vi "Main FK.vi"() -> ()   [LabVIEW 2017]
uses:
  <vilib>/Native 3D Graph/xcontrol/3DPC_SurfacePlot.xctl
  <vilib>/Native 3D Graph/classes/Line/Line.lvclass
  <vilib>/Platform/TimedLoop/XDataNode/timing_clust.ctl
  <vilib>/Platform/TimedLoop/XDataNode/nitl_modes.ctl
  <vilib>/Platform/TimedLoop/XDataNode/wakeup.ctl
  <vilib>/Analysis/Matrix/Datatypes/RealMatrix.ctl
  <vilib>/Utility/error.llb/DialogType.ctl
  <vilib>/Analysis/baseanly.llb/A x Vector.vi
  <vilib>/Analysis/baseanly.llb/Real A x B.vi
  <vilib>/Analysis/_algsub.llb/Vector Norm.vi
  <vilib>/Analysis/_algsub.llb/Real Vector Norm.vi
  <vilib>/Analysis/baseanly.llb/Outer Product.vi
  <vilib>/Analysis/baseanly.llb/Real Outer Product.vi
  <vilib>/robotics/Kinematics/Create Lie Group Matrix.vi
  <vilib>/Analysis/coordinate.llb/Direction Cosines To Euler Angles.vi
  <vilib>/Analysis/7linalg.llb/Create Special Matrix.vi
  <vilib>/Analysis/7linalg.llb/Create Special Real Matrix.vi
  <vilib>/Analysis/Matrix/Numeric/Multiply/Multiply.vi
  <vilib>/Analysis/Matrix/Numeric/Multiply/Multiply - RM,R.vi
  <vilib>/Analysis/Matrix/Numeric/Multiply/Multiply - R,RM.vi
  <vilib>/Analysis/Matrix/Numeric/Add/Add.vi
  <vilib>/Analysis/Matrix/Numeric/Add/Add - RM,RM.vi
  <vilib>/platform/TimedLoop/XDataNode/XDataNode.xnode
  <vilib>/robotics/Kinematics/NI_Kinematics.lvlib
  <vilib>/Analysis/NI_AALBase.lvlib
  <vilib>/Platform/TimedLoop/XDataNode/XDNodeRunTimeDep.lvlib
  <vilib>/Analysis/Matrix/NI_Matrix.lvlib
panel:
  out "FT":dbl[](array[numeric])
  out "w3c":dbl[](array[numeric])=[-0.5089191509681598, -0.8606888462607745, 0.014697200418595196]
  out "w1c":dbl[](array[numeric])=[0.9992375220058815, 0.022541625315148195, -0.031878672238615374]
  out "w2c":dbl[](array[numeric])=[-0.4945004015747698, 0.8691315050710928, 0.008931950248859025]
  out "u3":dbl[](array[numeric])=[-0.7071067811865474, 0.4082482904638634, -0.5773502691896257]
  out "u1":dbl[](array[numeric])=[0.0, -0.816496580927726, -0.5773502691896257]
  out "u2":dbl[](array[numeric])=[0.7071067811865476, 0.40824829046386285, -0.5773502691896257]
  in  "radius":dbl=1.0
  in  "damping":dbl[](array[numeric])=[0.5, 0.5, 0.5]
  out "3D Graph":refnum<class "Base Datatype.lvclass">[](xcontrol)
  in  "theta0":dbl[](array[numeric])=[0.0, 0.0, 0.0] format="%#_15g"
  in  "Kd":dbl=0.01 format="%#_13g"
  in  "Kp":dbl=10.0 format="%#_13g"
  out "thetac":dbl[](array[numeric])=[-0.03905316656235388, 0.010939578455381647, 0.018001293030222833] format="%#_15g"
  out "v3c":dbl[](array[numeric])=[0.5535037631925916, -0.3402635412966427, -0.7601672885595036]
  out "v1c":dbl[](array[numeric])=[-0.03873377001737612, 0.6749587725327184, -0.7368380761343479]
  out "v2c":dbl[](array[numeric])=[-0.6206923298860185, -0.34591671533767604, -0.7036211037701037]
  out "beta2":dbl=0.7460127831658564
  out "v30":dbl[](array[numeric])=[0.5877852522924729, -0.33935797363675174, -0.7344008870614411]
  out "v10":dbl[](array[numeric])=[0.0, 0.6787159472735029, -0.7344008870614411]
  out "v20":dbl[](array[numeric])=[-0.5877852522924731, -0.3393579736367513, -0.7344008870614411]
  out "dt":dbl=0.001
  in  "Period":i64=1
  out "v2d":dbl[](array[numeric])=[-0.6305174466734633, -0.34790000489268624, -0.6938395607314696]
  out "v1d":dbl[](array[numeric])=[-0.050680478981355706, 0.673803235637673, -0.7371707323913453]
  out "v3d":dbl[](array[numeric])=[0.5427020452710659, -0.34055660320835135, -0.7677862268039098]
  out "thetad":dbl[](array[numeric])=[-0.0511004594719751, 0.014220574258536452, 0.023656720268484584] format="%#_15g"
  out "message":string="No Error"
  out "error?":bool
  in  "stop":bool
  out "beta1":dbl=0.9553166181245093
  out "gamma2":dbl=1.2566370614359172
  out "gamma1":dbl=1.5707963267948966
  out "alpha2":dbl=1.5707963267948966
  out "alpha1":dbl=1.5707963267948966
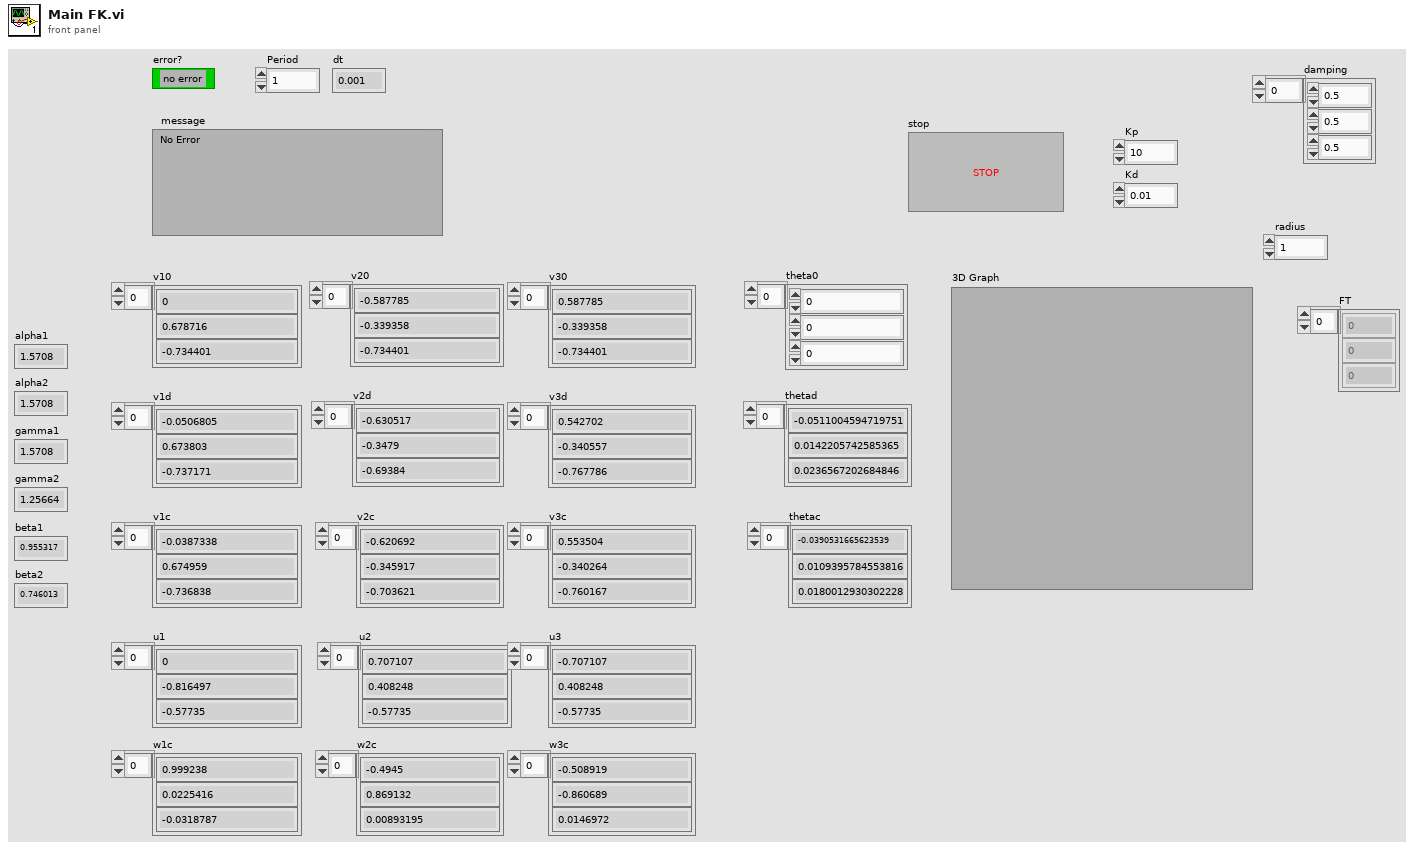
[diagram p1: front panel]
types:
  T1 = typedef "XDNodeRunTimeDep.lvlib/timing_clust.ctl" = cluster{"Expected End [f-1]":u64, "Actual End [f-1]":u64, "Finished Late? [f-1]":bool, "Expected End [i-1]":u64, "Actual End [i-1]":u64, "Finished Late? [i-1]":bool, "Expected Start [i]":u64, "Actual Start [i]":u64, "Expected Start [f]":u64, "Actual Start [f]":u64, "Source Name":string, "Structure Name":string, "Period":i64, "Deadline":i64, "Offset":i64, "Start":i64, "Priority":i32, "Timeout":i32, "Mode":T2, "Wakeup Reason":T3, "Error":errorcluster, "Source Type":string, "Secondary Source Type":string, "Global End Time":u64, "Global Start Time":u64, "Frame Duration":u64, "Iteration Duration":u64, "Assigned CPU":i32, "I/O Scan Engine Mode":u32}
  T2 = typedef "XDNodeRunTimeDep.lvlib/nitl_modes.ctl" = enum32{"No Change", "Process missed periods, maintain original phase", "Discard missed periods, maintain original phase", "Process missed periods, ignore original phase", "Discard missed periods, ignore original phase"}
  T3 = typedef "XDNodeRunTimeDep.lvlib/wakeup.ctl" = enum32{"Normal", "Aborted", "Asynchronous wakeup", "Timing source error", "Timed loop error", "Timeout"}
  T4 = typedef "NI_Matrix.lvlib/RealMatrix.ctl" = dbl[][]
  T5 = typedef "DialogType.ctl" = u16
  T6 = cluster{"phi (Z)":dbl, "theta (X)":dbl, "psi (Z)":dbl}
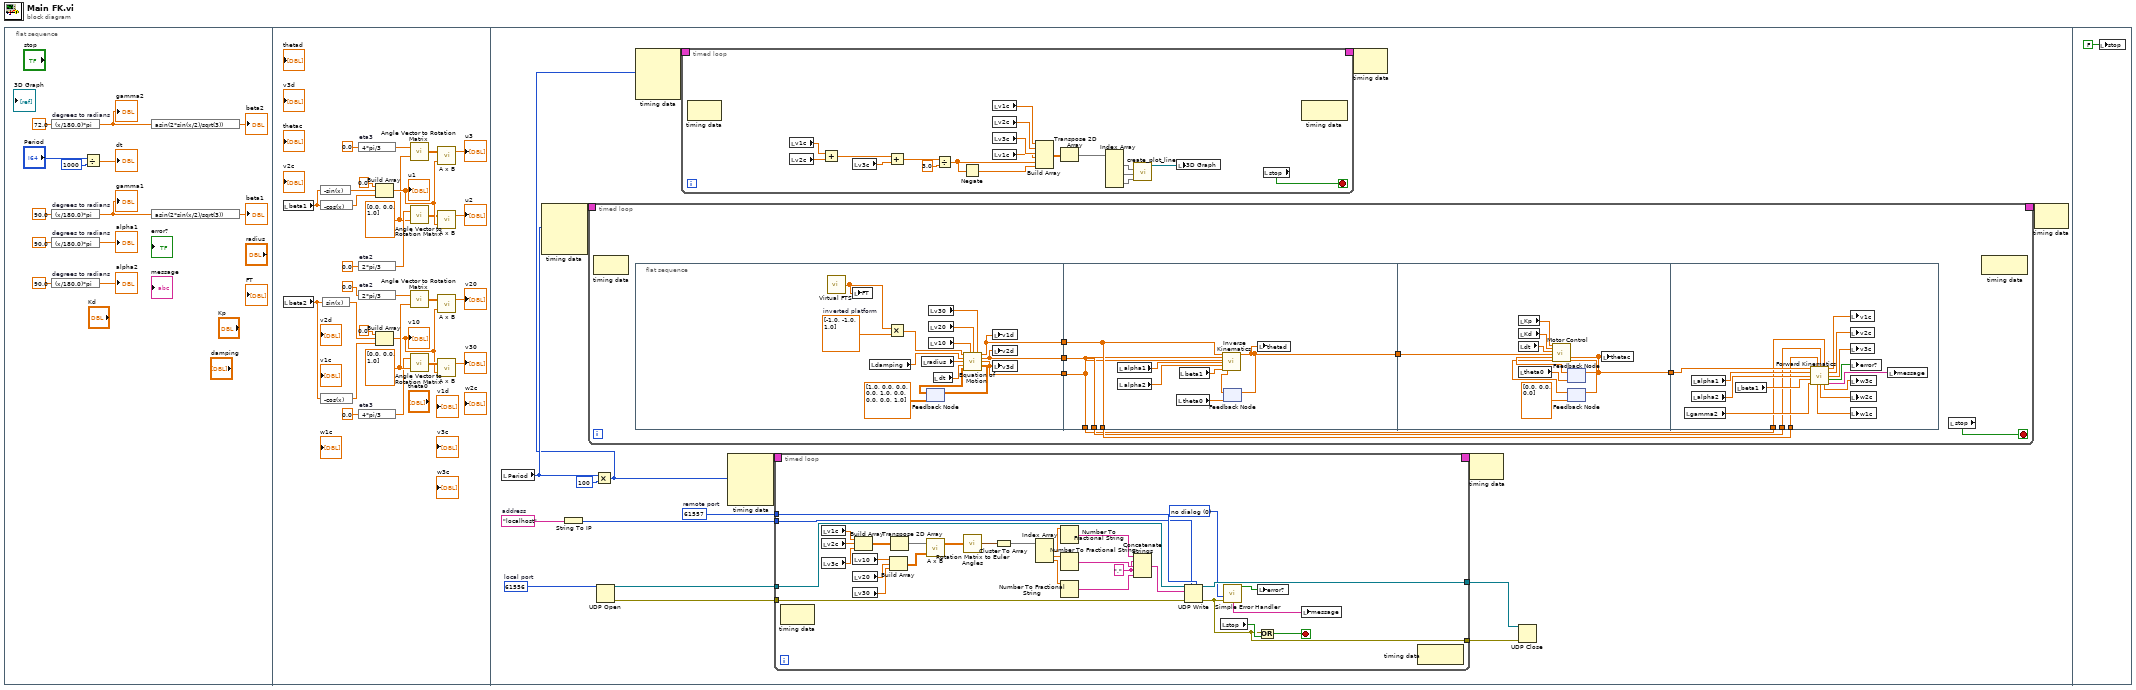
[diagram p0: block diagram]
diagram:
  n1 = flat-sequence {
    frame #0 {
      # "Design Parameters"
      n2 = expression code="(x/180.0)*pi" "degrees to radians"(72.0 ("gamma2")) -> (w5:dbl)
      "gamma2" <- w5
      n3 = expression code="(x/180.0)*pi" "degrees to radians"(90.0 ("gamma1")) -> (w7:dbl)
      "gamma1" <- w7
      n4 = expression code="(x/180.0)*pi" "degrees to radians"(90.0 ("alpha1")) -> (→"alpha1":dbl)
      n5 = expression code="(x/180.0)*pi" "degrees to radians"(90.0 ("alpha2")) -> (→"alpha2":dbl)
      n6 = Divide(x="Period", y=i64 1000) -> (x/y=→"dt":dbl)
      n7 = expression code="asin(2*sin(x/2)/sqrt(3))"(w5) -> (→"beta2":dbl)
      n8 = expression code="asin(2*sin(x/2)/sqrt(3))"(w7) -> (→"beta1":dbl)
    }
    frame #1 {
      w17 = dbl[] [0.0, 0.0, 1.0] ("vector")
      w38 = dbl[] [0.0, 0.0, 1.0] ("vector")
      # "Kinematics Variables"
      n9 = local read "beta1"() -> (w27:dbl)
      n10 = local read "beta2"() -> (w28:dbl)
      n11 = expression code="-cos(x)"(w27) -> (w16:dbl)
      n12 = expression code="-cos(x)"(w28) -> (w39:dbl)
      n13 = expression code="-sin(x)"(w27) -> (w15:dbl)
      n14 = expression code="sin(x)"(w28) -> (w40:dbl)
      n15 = expression code="4*pi/3" "eta3"(0.0) -> (w19:dbl)
      n16 = expression code="2*pi/3" "eta2"(0.0) -> (w18:dbl)
      n17 = expression code="2*pi/3" "eta2"(0.0) -> (w37:dbl)
      n18 = expression code="4*pi/3" "eta3"(0.0) -> (w36:dbl)
      n19 = Build Array(0.0 ("element"), w15, w16) -> (w24:dbl[])
      "u1" <- w24
      n20 = Build Array(0.0 ("element"), w40, w39) -> (w31:dbl[])
      "v10" <- w31
      n21 = call <vilib>:"Angle Vector to Rotation Matrix.vi"("vector"=w17, "angle"=w19) -> ("rotation matrix"=w21:T4)
      n22 = call <vilib>:"Angle Vector to Rotation Matrix.vi"("vector"=w17, "angle"=w18) -> ("rotation matrix"=w20:T4)
      n23 = call <vilib>:"Angle Vector to Rotation Matrix.vi"("vector"=w38, "angle"=w37) -> ("rotation matrix"=w35:T4)
      n24 = call <vilib>:"Angle Vector to Rotation Matrix.vi"("vector"=w38, "angle"=w36) -> ("rotation matrix"=w34:T4)
      n25 = call-poly <vilib>:"A x B.vi"("Vector"=w24, "A"=w21) -> ("A x Vector"=→"u3":dbl[])  [unwired: 1 out]
      n26 = call-poly <vilib>:"A x B.vi"("Vector"=w24, "A"=w20) -> ("A x Vector"=→"u2":dbl[])  [unwired: 1 out]
      n27 = call-poly <vilib>:"A x B.vi"("Vector"=w31, "A"=w35) -> ("A x Vector"=→"v20":dbl[])  [unwired: 1 out]
      n28 = call-poly <vilib>:"A x B.vi"("Vector"=w31, "A"=w34) -> ("A x Vector"=→"v30":dbl[])  [unwired: 1 out]
    }
    frame #2 {
      w51 = "localhost"  # address
      w52 = u16 61557  # remote port
      w49 = u16 61556  # local port
      # "FK/IK"
      n29 = local read "Period"() -> (w56:i64)
      n30 = node-c288(w56) -> (w58:T1)  [unwired: 3 in]
      n31 = String To IP(1:w51) -> (0:w50:u32)
      n32 = timed-loop {
        timing: w58 -> [_]
        timing-out: [_] -> w57
        stop <- w129 stop-if-true
        n33 = node-c288() -> ()  [unwired: 1 in, 1 out]
        n34 = flat-sequence {
          tunnel: [w135] -> w123
          tunnel: [w134] -> w122
          tunnel: [w133] -> w121
          tunnel: [w148] -> w128
          tunnel: [w147] -> w126
          tunnel: [w146] -> w125
          tunnel: [w145] -> w124
          tunnel: w123 -> [w147]
          tunnel: w122 -> [w146]
          tunnel: w121 -> [w145]
          tunnel: w128 -> [w155]
          tunnel: [w154] -> w127
          tunnel: w127 -> [w170]
          tunnel: w126 -> [w169]
          tunnel: w125 -> [w168]
          tunnel: w124 -> [w167]
          frame #0 {
            w131 = dbl[] [-1.0, -1.0, 1.0]  # inverted platform
            n35 = call "Virtual FTS.vi"() -> ("FT"=w130:dbl[])
            n36 = local write "FT"(w130) -> ()
            n37 = local read "damping"() -> (w144:dbl[])
            n38 = Multiply(x=w130, y=w131) -> (x*y=w132:dbl[])
            n39 = local read "radius"() -> (w143:dbl)
            n40 = feedback #1(T4 [[1.0, 0.0, 0.0], [0.0, 1.0, 0.0], [0.0, 0.0, 1.0]] ("R'")) -> (w140:T4)
            n41 = local read "v30"() -> (w136:dbl[])
            n42 = local read "v20"() -> (w137:dbl[])
            n43 = local read "v10"() -> (w138:dbl[])
            n44 = local read "dt"() -> (w142:dbl)
            n45 = call "Equation of Motion.vi"("FT"=w132, "v10"=w138, "v20"=w137, "v30"=w136, "damping"=w144, "radius"=w143, "dt"=w142, "R"=w140) -> ("v1d"=w135:dbl[], "v2d"=w134:dbl[], "v3d"=w133:dbl[], "R'"=w141:T4)  [unwired: 4 in]
            n46 = feedback-in #1(w141) -> ()
            n47 = local write "v1d"(w135) -> ()
            n48 = local write "v2d"(w134) -> ()
            n49 = local write "v3d"(w133) -> ()
          }
          frame #1 {
            n50 = local read "alpha1"() -> (w149:dbl)
            n51 = local read "alpha2"() -> (w150:dbl)
            n52 = local read "theta0"() -> (w152:dbl[])
            n53 = local read "beta1"() -> (w151:dbl)
            n54 = feedback #2(w152) -> (w153:dbl[])
            n55 = call "Inverse Kinematics.vi"("v1"=w147, "v2"=w146, "v3"=w145, "alpha1"=w149, "alpha2"=w150, "beta1"=w151, "theta"=w153) -> ("theta'"=w148:dbl[])  [unwired: 12 in]
            n56 = feedback-in #2(w148) -> ()
            n57 = local write "thetad"(w148) -> ()
          }
          frame #2 {
            n58 = local read "Kp"() -> (w163:dbl)
            n59 = local read "Kd"() -> (w162:dbl)
            n60 = local read "dt"() -> (w161:dbl)
            n61 = local read "theta0"() -> (w157:dbl[])
            n62 = feedback #3(w157) -> (w160:dbl[])
            n63 = feedback #4(dbl[] [0.0, 0.0, 0.0] ("e'")) -> (w158:dbl[])
            n64 = call "Motor Control.vi"("Kp"=w163, "Kd"=w162, "dt"=w161, "thetad"=w155, "thetac"=w160, "e"=w158) -> ("thetac'"=w154:dbl[], "e'"=w159:dbl[])  [unwired: 12 in]
            n65 = feedback-in #3(w154) -> ()
            n66 = feedback-in #4(w159) -> ()
            n67 = local write "thetac"(w154) -> ()
          }
          frame #3 {
            n68 = local read "gamma2"() -> (w174:dbl)
            n69 = local read "alpha1"() -> (w171:dbl)
            n70 = local read "alpha2"() -> (w172:dbl)
            n71 = local read "beta1"() -> (w173:dbl)
            n72 = call "Forward Kinematics.vi"("theta"=w170, "v1"=w169, "v2"=w168, "v3"=w167, "alpha1"=w171, "alpha2"=w172, "beta1"=w173, "gamma2"=w174) -> ("v1'"=w175:dbl[], "v2'"=w176:dbl[], "v3'"=w177:dbl[], "error?"=w179:bool, "w1c"=w166:dbl[], "w2c"=w165:dbl[], "w3c"=w164:dbl[], "message"=w178:string)
            n73 = local write "v1c"(w175) -> ()
            n74 = local write "v2c"(w176) -> ()
            n75 = local write "v3c"(w177) -> ()
            n76 = local write "error?"(w179) -> ()
            n77 = local write "w3c"(w164) -> ()
            n78 = local write "w2c"(w165) -> ()
            n79 = local write "w1c"(w166) -> ()
            n80 = local write "message"(w178) -> ()
          }
        }
        n81 = local read "stop"() -> (w129:bool)
        n82 = node-c288() -> ()  [unwired: 1 in, 1 out]
      }
      n83 = Multiply(x=w56, y=i64 100) -> (x*y=w42:i64)
      n84 = UDP Open(11:w49) -> (port=w48:refnum<k16>, 0:w46:errorcluster)  [unwired: 4 in, 1 out]
      n85 = node-c288(w42) -> (w44:T1)  [unwired: 3 in]
      n86 = timed-loop {
        timing: w44 -> [_]
        timing-out: [_] -> w43
        stop <- w59 stop-if-true
        n87 = node-c288() -> ()  [unwired: 1 in, 1 out]
        n88 = local read "v1c"() -> (w68:dbl[])
        n89 = local read "v2c"() -> (w67:dbl[])
        n90 = Add(x=w68, y=w67) -> (x+y=w66:dbl[])
        n91 = local read "v3c"() -> (w65:dbl[])
        n92 = Add(x=w66, y=w65) -> (x+y=w64:dbl[])
        n93 = Divide(x=w64, y=3.0) -> (x/y=w62:dbl[])
        n94 = Negate(x=w62) -> (-x=w61:dbl[])
        n95 = local read "v1c"() -> (w76:dbl[])
        n96 = local read "v2c"() -> (w75:dbl[])
        n97 = local read "v3c"() -> (w74:dbl[])
        n98 = local read "v1c"() -> (w73:dbl[])
        n99 = Build Array(w76, w75, w74, w73, w62, w61) -> (w72:dbl[][])
        n100 = Transpose 2D Array(2D array=w72) -> (transposed array=w71:dbl[][])
        n101 = Index Array(array=w71) -> (element #1=w70:dbl[], element #2=w69:dbl[], element #3=w60:dbl[])  [unwired: 6 in]
        n102 = call <vilib>:"create_plot_line.vi"("z vector"=w60, "y vector"=w69, "x vector"=w70) -> ("plots out"=w77:refnum<class "Base Datatype.lvclass">[])  [unwired: 2 in, 6 out]
        n103 = local write "3D Graph"(w77) -> ()
        n104 = local read "stop"() -> (w59:bool)
        n105 = node-c288() -> ()  [unwired: 1 in, 1 out]
      }
      n106 = node-c288(w42) -> (w54:T1)  [unwired: 3 in]
      n107 = timed-loop {
        timing: w54 -> [_]
        timing-out: [_] -> w53
        tunnel: w52 -> [w114]
        tunnel: w50 -> [w113]
        tunnel: w48 -> [w112]
        tunnel: [w111] -> w47
        tunnel: w46 -> [w110]
        tunnel: [w106] -> w45
        stop <- w108 stop-if-true
        w85 = "," ("string")
        w107 = T5 0 items=["no dialog", "OK message", "continue or stop message", "OK message + warnings", "continue/stop + warnings"] ("type of dialog (OK msg:1)")
        n108 = node-c288() -> ()  [unwired: 1 in, 1 out]
        n109 = local read "v1c"() -> (w103:dbl[])
        n110 = local read "v2c"() -> (w102:dbl[])
        n111 = local read "v3c"() -> (w101:dbl[])
        n112 = local read "v10"() -> (w98:dbl[])
        n113 = local read "v20"() -> (w99:dbl[])
        n114 = local read "v30"() -> (w100:dbl[])
        n115 = Build Array(w103, w102, w101) -> (w97:dbl[][])
        n116 = Build Array(w98, w99, w100) -> (w95:dbl[][])
        n117 = Transpose 2D Array(2D array=w97) -> (transposed array=w96:dbl[][])
        n118 = call-poly <vilib>:"A x B.vi"("B"=w95, "A"=w96) -> ("A x B"=w94:T4)  [unwired: 1 out]
        n119 = call <vilib>:"Rotation Matrix to Euler Angles.vi"("rotation matrix"=w94) -> ("euler angles"=w93:T6)
        n120 = Cluster To Array(cluster=w93) -> (array=w92:dbl[])
        n121 = Index Array(array=w92) -> (element #1=w91:dbl, element #2=w90:dbl, element #3=w89:dbl)  [unwired: 3 in]
        n122 = Number To Fractional String(number=w91) -> (F-format string=w88:string)  [unwired: 3 in]
        n123 = Number To Fractional String(number=w90) -> (F-format string=w87:string)  [unwired: 3 in]
        n124 = Number To Fractional String(number=w89) -> (F-format string=w86:string)  [unwired: 3 in]
        n125 = Concatenate Strings(w88, w85, w87, w85, w86) -> (w84:string)
        n126 = UDP Write(address=w113, port or service name=w114, connection ID=w112, data in=w84, 8:w110) -> (error out=w106:errorcluster, 3:w111:refnum<k16>)  [unwired: 1 in]
        n127 = local read "stop"() -> (w109:bool)
        n128 = call <vilib>:"Simple Error Handler.vi"("type of dialog (OK msg:1)"=w107, "error in (no error)"=w106) -> ("error?"=w105:bool, "message"=w104:string)  [unwired: 3 in, 3 out]
        n129 = local write "error?"(w105) -> ()
        n130 = Or(x=w106, y=w109) -> (x .or. y?=w108:bool)
        n131 = local write "message"(w104) -> ()
        n132 = node-c288() -> ()  [unwired: 1 in, 1 out]
      }
      n133 = node-c288(w43) -> ()  [unwired: 1 out]
      n134 = node-c288(w53) -> ()  [unwired: 1 out]
      n135 = UDP Close(connection ID=w47, 8:w45) -> ()  [unwired: 2 out]
      n136 = node-c288(w57) -> ()  [unwired: 1 out]
    }
    frame #3 {
      n137 = local write "stop"(FALSE ("stop")) -> ()
    }
  }
